vi "Empty RX buffer.vi"(8 "error in (no error)":errorcluster, 11 "RP Transceiver in":refnum<class "RP Transceiver.lvclass">) -> (0 "error out":errorcluster, 2 "Data out":i32[](array[numeric]), 3 "RP Transceiver out":refnum<class "RP Transceiver.lvclass">)   [LabVIEW 2015, in "RP Transceiver.lvclass"]
uses:
  RP Transceiver.lvclass
  RP Transceiver.lvclass/RP Transceiver.ctl
  RP Communicator/RP Communicator.lvclass
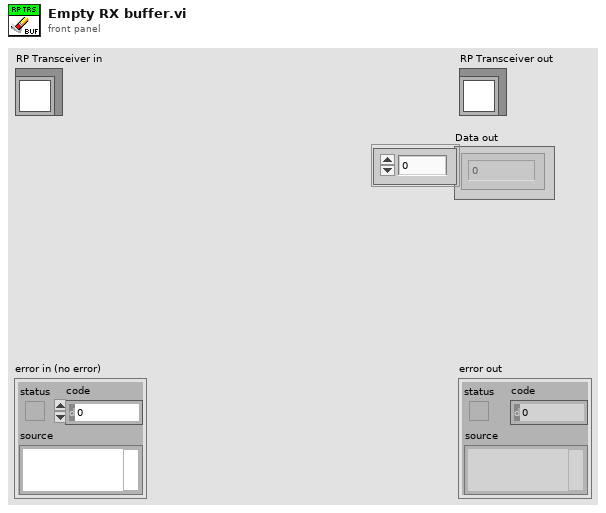
[diagram p1: front panel]
types:
  T1 = typedef "Receiver format.ctl" = enum16{"X-Y-F", "F-X-Y", "X-Y", "X"}
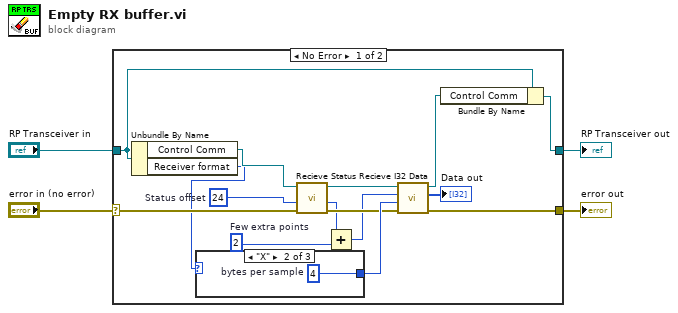
[diagram p0: block diagram]
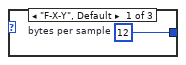
[diagram p2: hidden frame]
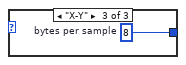
[diagram p3: hidden frame]
diagram:
  n1 = case shown="No Error" "error in (no error)" {
    selector: "error in (no error)" -> [w12 w24]
    tunnel: [w11 w24] -> w3
    tunnel: [w18 w23] -> w1
    tunnel: "RP Transceiver in" -> [w19 w23]
    frame No Error {
      w6 = u32 2  # Few extra points
      w17 = u64 24  # Status offset
      n2 = Unbundle By Name(w19) -> ("Control Comm"=w16:refnum<class "RP Communicator.lvclass">, "Receiver format"=w5:T1)
      n3 = case shown="\"X\"" w5 {
        tunnel: [w20 w21 w22] -> w15
        frame "F-X-Y", Default {
          w20 = 12  # bytes per sample
        }
        frame "X" {
          w21 = 4  # bytes per sample
        }
        frame "X-Y" {
          w22 = 8  # bytes per sample
        }
      }
      n4 = call-dynamic "Recieve Status.vi"("error in (no error)"=w12, "Status offset"=w17, "RP Communicator in"=w16) -> ("error out"=w13:errorcluster, "Status response"=w7:u32, "RP Communicator out"=w14:refnum<class "RP Communicator.lvclass">)  [unwired: 6 in]
      n5 = Add(x=w7, y=w6) -> (x+y=w8:u32)
      n6 = call-dynamic "Recieve I32 Data.vi"("error in (no error)"=w13, "bytes per sample"=w15, "Samples per read"=w8, "RP Communicator in"=w14) -> ("error out"=w11:errorcluster, "Data out"=→"Data out":i32[], "RP Communicator out"=w9:refnum<class "RP Communicator.lvclass">)  [unwired: 5 in]
      n7 = Bundle By Name(cluster=w19, "Control Comm"=w9) -> (w18:refnum<class "RP Transceiver.lvclass">)
    }
    frame Error {
    }
  }
  "error out" <- w3
  "RP Transceiver out" <- w1
